vi "Logger.Variant.Read.vi"(8 "error in (no error)":errorcluster, 11 "VariantSets in":T2={"State"=enum."Init", "ImgPath"=path "", "WabcoPlate"="", "WabcoProduct"="", "ClientProduct"="", "ClientPlate"="", "TotalQuantity"=0, "OrderQuantity"=0, "Serial"=0, "Wabco"={"LaserJob"="", "AdditionalTxt"="037", "FactoryCode"="", "RevID"=0, "ForkID"=0, "FailuresLimit"=0, "GlobalCnt"=0, "ScannerProgram"=0, "SerialFormat"=enum."6 dig", "CoordA"={"X"=0.0, "Y"=0.0, "Angle"=0.0}, "CoordB"={"X"=0.0, "Y"=0.0, "Angle"=0.0}, "DMCconfig"=0, "CVX_Program"=0}, "Client"={"LaserJob"="", "AdditionalTxt"="", "FactoryCode"="037", "RevID"=0, "ForkID"=0, "FailuresLimit"=0, "GlobalCnt"=0, "ScannerProgram"=0, "SerialFormat"=enum."6 dig", "CoordA"={"X"=0.0, "Y"=0.0, "Angle"=0.0}, "CoordB"={"X"=0.0, "Y"=0.0, "Angle"=0.0}, "DMCconfig"=0, "CVX_Program"=0}}) -> (0 "error out":errorcluster, 1 "ClientPlateImg":picture, 2 "WabcoPlateImg":picture, 3 "VariantSets out":T2={"State"=enum."Init", "ImgPath"=path "", "WabcoPlate"="", "WabcoProduct"="", "ClientProduct"="", "ClientPlate"="", "TotalQuantity"=0, "OrderQuantity"=0, "Serial"=0, "Wabco"={"LaserJob"="", "AdditionalTxt"="037", "FactoryCode"="", "RevID"=0, "ForkID"=0, "FailuresLimit"=0, "GlobalCnt"=0, "ScannerProgram"=0, "SerialFormat"=enum."6 dig", "CoordA"={"X"=0.0, "Y"=0.0, "Angle"=0.0}, "CoordB"={"X"=0.0, "Y"=0.0, "Angle"=0.0}, "DMCconfig"=0, "CVX_Program"=0}, "Client"={"LaserJob"="", "AdditionalTxt"="", "FactoryCode"="037", "RevID"=0, "ForkID"=0, "FailuresLimit"=0, "GlobalCnt"=0, "ScannerProgram"=0, "SerialFormat"=enum."6 dig", "CoordA"={"X"=0.0, "Y"=0.0, "Angle"=0.0}, "CoordB"={"X"=0.0, "Y"=0.0, "Angle"=0.0}, "DMCconfig"=0, "CVX_Program"=0}}, 5 "OrdersTableIdx":i32, 7 "OrdersTable":string[][](array[string]))   [LabVIEW 2016]
uses:
  Logger.Variant.Sets.ctl
  Station/Station.Changeover.State.vi
  Station/Station.Plate.Properties.ctl
  Sequence/Sequence.Code.SerialFormat.ctl
  Drivers/V7310/LowLevel/V7310.Job.Sets.ctl
  Global/ApplicationGlobal.vi
  Drivers/V7310/LowLevel/V7310.Global.vi
panel:
  in  "SerialFormat":T1
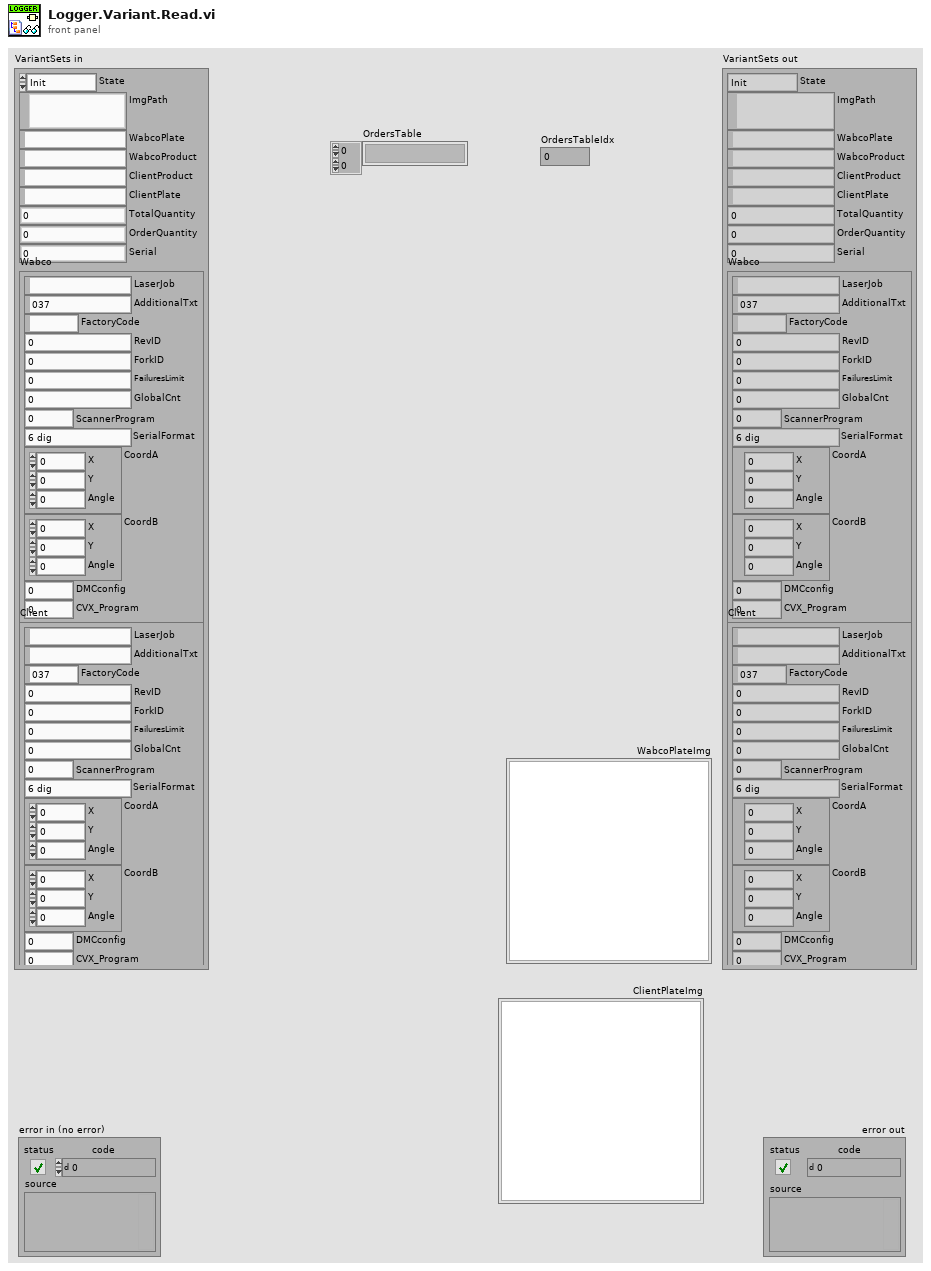
[diagram p1: front panel]
types:
  T1 = typedef "Sequence.Code.SerialFormat.ctl" = enum8{"", "6 dig", "7 dig"}
  T2 = typedef "Logger.Variant.Sets.ctl" = cluster{"State":T3, "ImgPath":path, "WabcoPlate":string, "WabcoProduct":string, "ClientProduct":string, "ClientPlate":string, "TotalQuantity":u16, "OrderQuantity":u16, "Serial":i32, "Wabco":T4, "Client":T4}
  T3 = typedef "Station.Changeover.State.vi" = enum16{"Init", "Scaning", "NOK", "Wait for ack", "Ready"}
  T4 = typedef "Station.Plate.Properties.ctl" = cluster{"LaserJob":string, "AdditionalTxt":string, "FactoryCode":string, "RevID":u8, "ForkID":u8, "FailuresLimit":u16, "GlobalCnt":i32, "ScannerProgram":u8, "SerialFormat":T1, "CoordA":T5, "CoordB":T5, "DMCconfig":i32, "CVX_Program":u16}
  T5 = typedef "V7310.Job.Sets.ctl" = cluster{"X":dbl, "Y":dbl, "Angle":dbl}
  T6 = cluster{"WabcoPlate":string, "WabcoProduct":string, "ClientProduct":string, "ClientPlate":string}
  T7 = typedef "imagedata.ctl" = cluster{"image type":i32, "image depth":i32, "image":u8[], "mask":u8[], "colors":u32[], "Rectangle":cluster{"left":i16, "top":i16, "right":i16, "bottom":i16}}
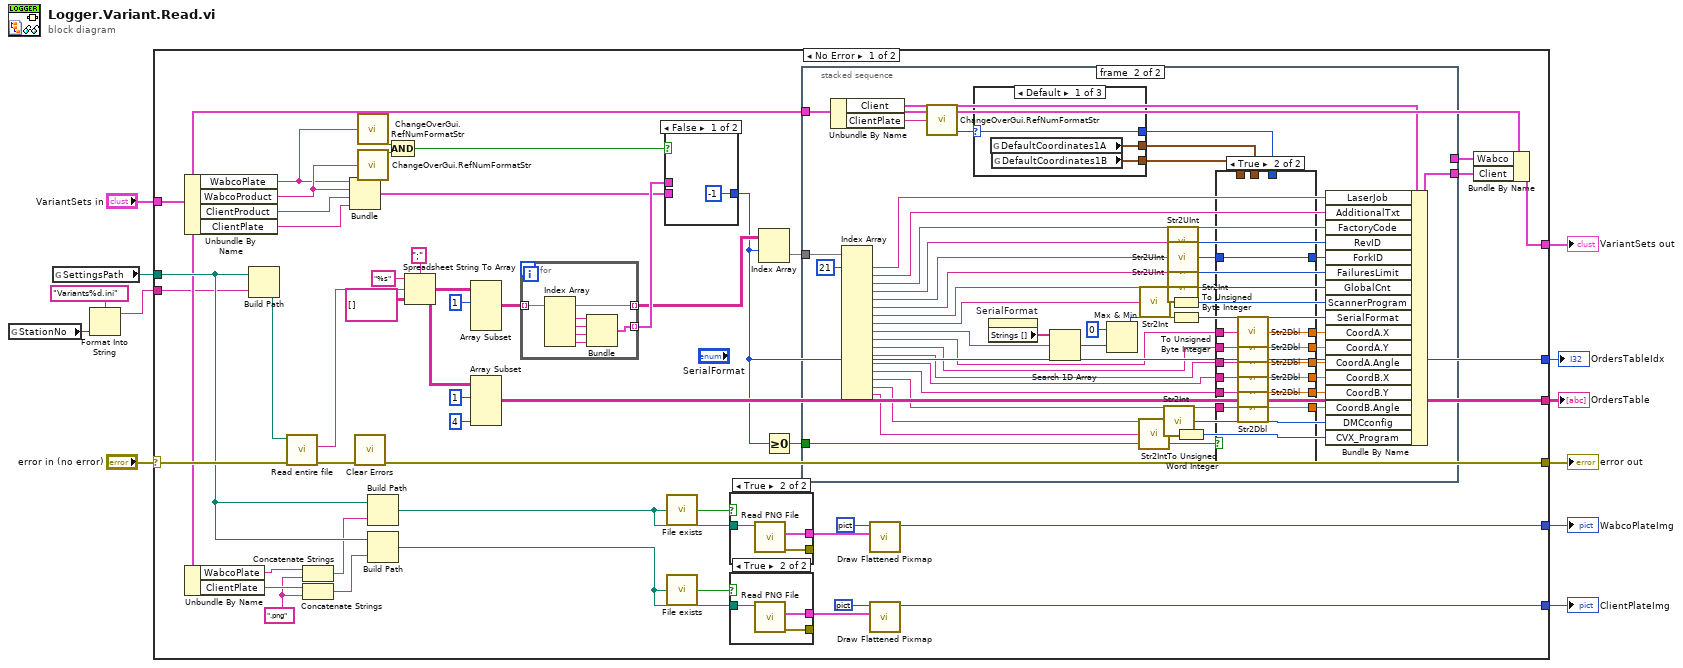
[diagram p0: block diagram]
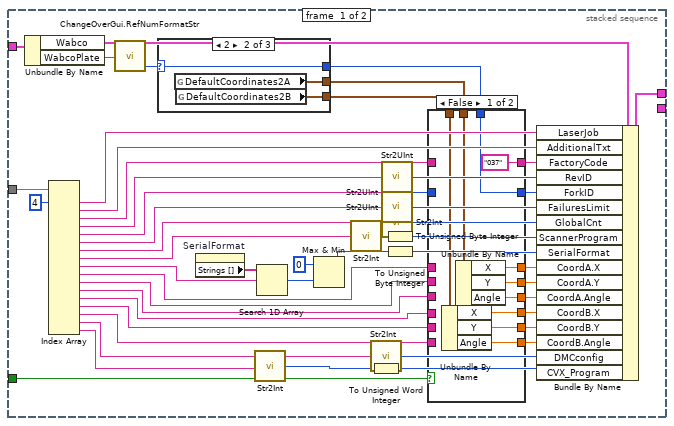
[diagram p2: hidden frame]
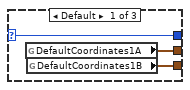
[diagram p3: hidden frame]
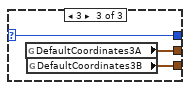
[diagram p4: hidden frame]
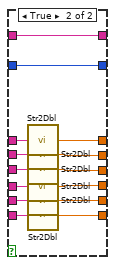
[diagram p5: hidden frame]
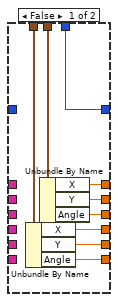
[diagram p6: hidden frame]
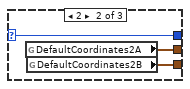
[diagram p7: hidden frame]
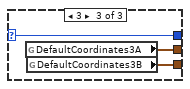
[diagram p8: hidden frame]
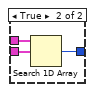
[diagram p9: hidden frame]
diagram:
  n1 = global read "ApplicationGlobal.vi" "StationNo"() -> (w2:i32)
  n2 = global read "ApplicationGlobal.vi" "SettingsPath"() -> (w10:path)
  n3 = Format Into String(format string="Variants%d.ini", w2) -> (resulting string=w1:string)  [unwired: 2 in, 1 out]
  n4 = case shown="No Error" "error in (no error)" {
    selector: "error in (no error)" -> [w59 w240]
    tunnel: [w28 w240] -> w11
    tunnel: w10 -> [w50 _]
    tunnel: [w24 _] -> w8
    tunnel: [w60 _] -> w9
    tunnel: "VariantSets in" -> [w16 _]
    tunnel: [w39 _] -> w6
    tunnel: [w17 _] -> w5
    tunnel: [w15 _] -> w4
    tunnel: w1 -> [w13 _]
    frame No Error {
      w46 = ".png" ("string")
      n5 = Unbundle By Name(w16) -> ("WabcoPlate"=w30:string, "WabcoProduct"=w31:string, "ClientProduct"=w37:string, "ClientPlate"=w21:string)
      n6 = Unbundle By Name(w16) -> ("WabcoPlate"=w47:string, "ClientPlate"=w49:string)
      n7 = Build Path(base path=w50, name or relative path=w13) -> (appended path=w55:path)
      n8 = call "Read entire file.vi"("error in"=w59, "file"=w55) -> ("error out"=w34:errorcluster, "contents"=w54:string)  [unwired: 4 in]
      n9 = Concatenate Strings(w47, w46) -> (w45:string)
      n10 = Concatenate Strings(w49, w46) -> (w48:string)
      n11 = Bundle("WabcoPlate"=w30, "WabcoProduct"=w31, "ClientProduct"=w37, "ClientPlate"=w21) -> (w35:T6)  [unwired: 1 in]
      n12 = call <vilib>:"Clear Errors.vi"("error in (no error)"=w34) -> ("error out"=w28:errorcluster)  [unwired: 5 in, 1 out]
      n13 = call "ChangeOverGui.RefNumFormatStr.vi"("RefNum in"=w30) -> ("RefNum format ok?"=w33:bool)  [unwired: 2 out]
      n14 = call "ChangeOverGui.RefNumFormatStr.vi"("RefNum in"=w31) -> ("RefNum format ok?"=w32:bool)  [unwired: 2 out]
      n15 = Build Path(base path=w50, name or relative path=w45) -> (appended path=w44:path)
      n16 = Build Path(base path=w50, name or relative path=w48) -> (appended path=w40:path)
      n17 = Compound Arithmetic op=AND(w33, w32) -> (w29:bool)
      n18 = Spreadsheet String To Array(delimiter (Tab)=";", format string="%s", spreadsheet string=w54, array type (2D Dbl)=string[][] []) -> (array=w20:string[][])
      n19 = Array Subset(array=w20, index (row)=1 ("index")) -> (w27:string[][])  [unwired: 3 in]
      n20 = Array Subset(array=w20, index (row)=1 ("index"), length (col)=4 ("length")) -> (w17:string[][])  [unwired: 2 in]
      n21 = for {
        tunnel: w27 -> [w225] mode=indexing
        tunnel: [w226] -> w36 mode=indexing
        tunnel: [w225] -> w26 mode=indexing
        n22 = Index Array(array=w225) -> (element #1=w229:string, element #2=w228:string, element #3=w227:string, element #4=w224:string)  [unwired: 4 in]
        n23 = Bundle(w229, w228, w227, w224) -> (w226:cluster{string, string, string, string})  [unwired: 1 in]
      }
      n24 = case shown="False" w29 {
        tunnel: w36 -> [_ w233]
        tunnel: w35 -> [_ w232]
        tunnel: [-1 ("index of element") w231] -> w15
        frame False {
        }
        frame True {
          n25 = Search 1D Array(1D array=w233, element=w232) -> (index of element=w231:i32)  [unwired: 1 in]
        }
      }
      n26 = call "File exists.vi"("file path"=w44) -> ("exists?"=w58:bool)  [unwired: 4 in]
      n27 = call "File exists.vi"("file path"=w40) -> ("exists?"=w41:bool)  [unwired: 4 in]
      n28 = case shown="True" w58 {
        tunnel: w44 -> [_ w239]
        tunnel: [_ w238] -> w56
        tunnel: [_ w237] -> _
        frame False {
        }
        frame True {
          n29 = call <vilib>:"Read PNG File.vi"("path to PNG file"=w239) -> ("error out"=w237:errorcluster, "image data"=w238:T7)  [unwired: 8 in, 1 out]
        }
      }
      n30 = case shown="True" w41 {
        tunnel: w40 -> [_ w236]
        tunnel: [_ w235] -> w43
        tunnel: [_ w234] -> _
        frame False {
        }
        frame True {
          n31 = call <vilib>:"Read PNG File.vi"("path to PNG file"=w236) -> ("error out"=w234:errorcluster, "image data"=w235:T7)  [unwired: 8 in, 1 out]
        }
      }
      n32 = Index Array(array=w26, index (row)=w15) -> (element=w25:string[])  [unwired: 1 in]
      n33 = Greater Or Equal To 0?(x=w15) -> (x >= 0?=w14:bool)
      n34 = stacked-sequence {
        tunnel: w25 -> [w108 w190]
        tunnel: w16 -> [w80 w172]
        tunnel: [w106 _] -> w23
        tunnel: [_ w173] -> w22
        tunnel: w14 -> [w79 w169]
        frame #0 {
          n35 = Unbundle By Name(w80) -> ("Wabco"=w110:T4, "WabcoPlate"=w78:string)
          n36 = Index Array(array=w108, index #1=4 ("index")) -> (element #1=w107:string, element #2=w105:string, element #3=w74:string, element #4=w103:string, element #5=w66:string, element #6=w101:string, element #7=w99:string, element #8=w64:string, element #9=w87:string, element #10=w86:string, element #11=w85:string, element #12=w84:string, element #13=w83:string, element #14=w82:string, element #15=w81:string, element #16=w70:string, element #17=w63:string)  [unwired: 16 in]
          n37 = call "ChangeOverGui.RefNumFormatStr.vi"("RefNum in"=w78) -> ("Idx"=w77:i32)  [unwired: 2 out]
          n38 = case shown="2" w77 {
            selector: w77 -> [w111 w114 w117]
            tunnel: [w113 w116 w119] -> w76
            tunnel: [w112 w115 w118] -> w75
            tunnel: [w111 w114 w117] -> w72
            frame Default {
              n39 = global read "V7310.Global.vi" "DefaultCoordinates1A"() -> (w113:T5)
              n40 = global read "V7310.Global.vi" "DefaultCoordinates1B"() -> (w112:T5)
            }
            frame 2 {
              n41 = global read "V7310.Global.vi" "DefaultCoordinates2A"() -> (w116:T5)
              n42 = global read "V7310.Global.vi" "DefaultCoordinates2B"() -> (w115:T5)
            }
            frame 3 {
              n43 = global read "V7310.Global.vi" "DefaultCoordinates3A"() -> (w119:T5)
              n44 = global read "V7310.Global.vi" "DefaultCoordinates3B"() -> (w118:T5)
            }
          }
          n45 = property on="SerialFormat" class="Enum (strict)"() -> ("Strings []"=w98:string[])  [unwired: 2 in, 2 out]
          n46 = call "Str2Int.vi"("string"=w63) -> ("Numeric"=w62:i32)
          n47 = Search 1D Array(1D array=w98, element=w87) -> (index of element=w97:i32)  [unwired: 1 in]
          n48 = Max & Min(x=0, y=w97) -> (max(x,y)=w94:i32)  [unwired: 1 out]
          n49 = call "Str2Int.vi"("string"=w64) -> ("Numeric"=w67:i32)
          n50 = call "Str2Int.vi"("string"=w70) -> ("Numeric"=w69:i32)
          n51 = To Unsigned Word Integer(number=w62) -> (unsigned 16bit integer=w61:u16)
          n52 = call "Str2UInt.vi"("string"=w103) -> ("Numeric"=w104:u32)
          n53 = call "Str2UInt.vi"("string"=w66) -> ("Numeric"=w65:u32)
          n54 = call "Str2UInt.vi"("string"=w101) -> ("Numeric"=w102:u32)
          n55 = call "Str2Int.vi"("string"=w99) -> ("Numeric"=w100:i32)
          n56 = To Unsigned Byte Integer(number=w67) -> (unsigned 8bit integer=w68:u8)
          n57 = To Unsigned Byte Integer(number=w94) -> (unsigned 8bit integer=w95:u8)
          n58 = case shown="False" w79 {
            tunnel: [w128 w143] -> w93
            tunnel: [w127 w142] -> w92
            tunnel: [w126 w141] -> w91
            tunnel: [w124 w140] -> w90
            tunnel: [w123 w139] -> w89
            tunnel: [w122 w138] -> w88
            tunnel: w86 -> [_ w137]
            tunnel: w85 -> [_ w136]
            tunnel: w84 -> [_ w135]
            tunnel: w83 -> [_ w134]
            tunnel: w82 -> [_ w133]
            tunnel: w81 -> [_ w132]
            tunnel: w76 -> [w129 _]
            tunnel: w75 -> [w125 _]
            tunnel: w74 -> [_ w131]
            tunnel: ["037" w131] -> w73
            tunnel: w72 -> [w120 _]
            tunnel: [w120 w130] -> w71
            tunnel: w65 -> [_ w130]
            frame False {
              n59 = Unbundle By Name(w125) -> ("X"=w124:dbl, "Y"=w123:dbl, "Angle"=w122:dbl)
              n60 = Unbundle By Name(w129) -> ("X"=w128:dbl, "Y"=w127:dbl, "Angle"=w126:dbl)
            }
            frame True {
              n61 = call "Str2Dbl.vi"("string"=w137) -> ("Numeric"=w143:dbl)
              n62 = call "Str2Dbl.vi"("string"=w136) -> ("Numeric"=w142:dbl)
              n63 = call "Str2Dbl.vi"("string"=w135) -> ("Numeric"=w141:dbl)
              n64 = call "Str2Dbl.vi"("string"=w134) -> ("Numeric"=w140:dbl)
              n65 = call "Str2Dbl.vi"("string"=w133) -> ("Numeric"=w139:dbl)
              n66 = call "Str2Dbl.vi"("string"=w132) -> ("Numeric"=w138:dbl)
            }
          }
          n67 = Bundle By Name(cluster=w110, "LaserJob"=w107, "AdditionalTxt"=w105, "FactoryCode"=w73, "RevID"=w104, "ForkID"=w71, "FailuresLimit"=w102, "GlobalCnt"=w100, "ScannerProgram"=w68, "SerialFormat"=w95, "CoordA.X"=w93, "CoordA.Y"=w92, "CoordA.Angle"=w91, "CoordB.X"=w90, "CoordB.Y"=w89, "CoordB.Angle"=w88, "DMCconfig"=w69, "CVX_Program"=w61) -> (w106:T4)
        }
        frame #1 {
          n68 = Unbundle By Name(w172) -> ("Client"=w192:T4, "ClientPlate"=w170:string)
          n69 = Index Array(array=w190, index #1=21 ("index")) -> (element #1=w189:string, element #2=w188:string, element #3=w187:string, element #4=w185:string, element #5=w184:string, element #6=w182:string, element #7=w180:string, element #8=w147:string, element #9=w174:string, element #10=w166:string, element #11=w165:string, element #12=w164:string, element #13=w167:string, element #14=w168:string, element #15=w163:string, element #16=w151:string, element #17=w146:string)  [unwired: 16 in]
          n70 = call "ChangeOverGui.RefNumFormatStr.vi"("RefNum in"=w170) -> ("Idx"=w171:i32)  [unwired: 2 out]
          n71 = case shown="Default" w171 {
            selector: w171 -> [w215 w218 w221]
            tunnel: [w217 w220 w223] -> w162
            tunnel: [w216 w219 w222] -> w161
            tunnel: [w215 w218 w221] -> w153
            frame Default {
              n72 = global read "V7310.Global.vi" "DefaultCoordinates1A"() -> (w217:T5)
              n73 = global read "V7310.Global.vi" "DefaultCoordinates1B"() -> (w216:T5)
            }
            frame 2 {
              n74 = global read "V7310.Global.vi" "DefaultCoordinates2A"() -> (w220:T5)
              n75 = global read "V7310.Global.vi" "DefaultCoordinates2B"() -> (w219:T5)
            }
            frame 3 {
              n76 = global read "V7310.Global.vi" "DefaultCoordinates3A"() -> (w223:T5)
              n77 = global read "V7310.Global.vi" "DefaultCoordinates3B"() -> (w222:T5)
            }
          }
          n78 = property on="SerialFormat" class="Enum (strict)"() -> ("Strings []"=w179:string[])  [unwired: 2 in, 2 out]
          n79 = Search 1D Array(1D array=w179, element=w174) -> (index of element=w178:i32)  [unwired: 1 in]
          n80 = Max & Min(x=0, y=w178) -> (max(x,y)=w175:i32)  [unwired: 1 out]
          n81 = call "Str2Int.vi"("string"=w146) -> ("Numeric"=w145:i32)
          n82 = call "Str2Int.vi"("string"=w147) -> ("Numeric"=w148:i32)
          n83 = call "Str2Int.vi"("string"=w151) -> ("Numeric"=w150:i32)
          n84 = call "Str2UInt.vi"("string"=w185) -> ("Numeric"=w186:u32)
          n85 = call "Str2UInt.vi"("string"=w184) -> ("Numeric"=w152:u32)
          n86 = call "Str2UInt.vi"("string"=w182) -> ("Numeric"=w183:u32)
          n87 = call "Str2Int.vi"("string"=w180) -> ("Numeric"=w181:i32)
          n88 = To Unsigned Byte Integer(number=w148) -> (unsigned 8bit integer=w149:u8)
          n89 = To Unsigned Byte Integer(number=w175) -> (unsigned 8bit integer=w176:u8)
          n90 = To Unsigned Word Integer(number=w145) -> (unsigned 16bit integer=w144:u16)
          n91 = case shown="True" w169 {
            tunnel: [w200 w214] -> w160
            tunnel: [w199 w213] -> w159
            tunnel: [w198 w212] -> w158
            tunnel: [w196 w211] -> w157
            tunnel: [w195 w210] -> w156
            tunnel: [w194 w209] -> w155
            tunnel: w162 -> [w201 _]
            tunnel: w161 -> [w197 _]
            tunnel: w168 -> [_ w208]
            tunnel: w167 -> [_ w207]
            tunnel: w166 -> [_ w206]
            tunnel: w165 -> [_ w205]
            tunnel: w164 -> [_ w204]
            tunnel: w163 -> [_ w203]
            tunnel: [w193 w202] -> w154
            tunnel: w153 -> [w193 _]
            tunnel: w152 -> [_ w202]
            frame False {
              n92 = Unbundle By Name(w197) -> ("X"=w196:dbl, "Y"=w195:dbl, "Angle"=w194:dbl)
              n93 = Unbundle By Name(w201) -> ("X"=w200:dbl, "Y"=w199:dbl, "Angle"=w198:dbl)
            }
            frame True {
              n94 = call "Str2Dbl.vi"("string"=w206) -> ("Numeric"=w214:dbl)
              n95 = call "Str2Dbl.vi"("string"=w205) -> ("Numeric"=w213:dbl)
              n96 = call "Str2Dbl.vi"("string"=w204) -> ("Numeric"=w212:dbl)
              n97 = call "Str2Dbl.vi"("string"=w207) -> ("Numeric"=w211:dbl)
              n98 = call "Str2Dbl.vi"("string"=w208) -> ("Numeric"=w210:dbl)
              n99 = call "Str2Dbl.vi"("string"=w203) -> ("Numeric"=w209:dbl)
            }
          }
          n100 = Bundle By Name(cluster=w192, "LaserJob"=w189, "AdditionalTxt"=w188, "FactoryCode"=w187, "RevID"=w186, "ForkID"=w154, "FailuresLimit"=w183, "GlobalCnt"=w181, "ScannerProgram"=w149, "SerialFormat"=w176, "CoordA.X"=w160, "CoordA.Y"=w159, "CoordA.Angle"=w158, "CoordB.X"=w157, "CoordB.Y"=w156, "CoordB.Angle"=w155, "DMCconfig"=w150, "CVX_Program"=w144) -> (w173:T4)
        }
      }
      n101 = call <vilib>:"Draw Flattened Pixmap.vi"("image data"=w56, "picture"=picture data[5B]) -> ("new picture"=w60:picture)  [unwired: 7 in]
      n102 = call <vilib>:"Draw Flattened Pixmap.vi"("image data"=w43, "picture"=picture data[5B]) -> ("new picture"=w39:picture)  [unwired: 7 in]
      n103 = Bundle By Name(cluster=w16, "Wabco"=w23, "Client"=w22) -> (w24:T2)
    }
    frame Error {
    }
  }
  "error out" <- w11
  "WabcoPlateImg" <- w9
  "VariantSets out" <- w8
  "ClientPlateImg" <- w6
  "OrdersTable" <- w5
  "OrdersTableIdx" <- w4
